vi "acquireVolumeAndFindNeurons.vi"   [LabVIEW 2017]
uses:
  globalUtilities.vi
  globalDevices.vi
  <userlib>/Hamamatsu Video Capture/tm_getframe16_40.vi
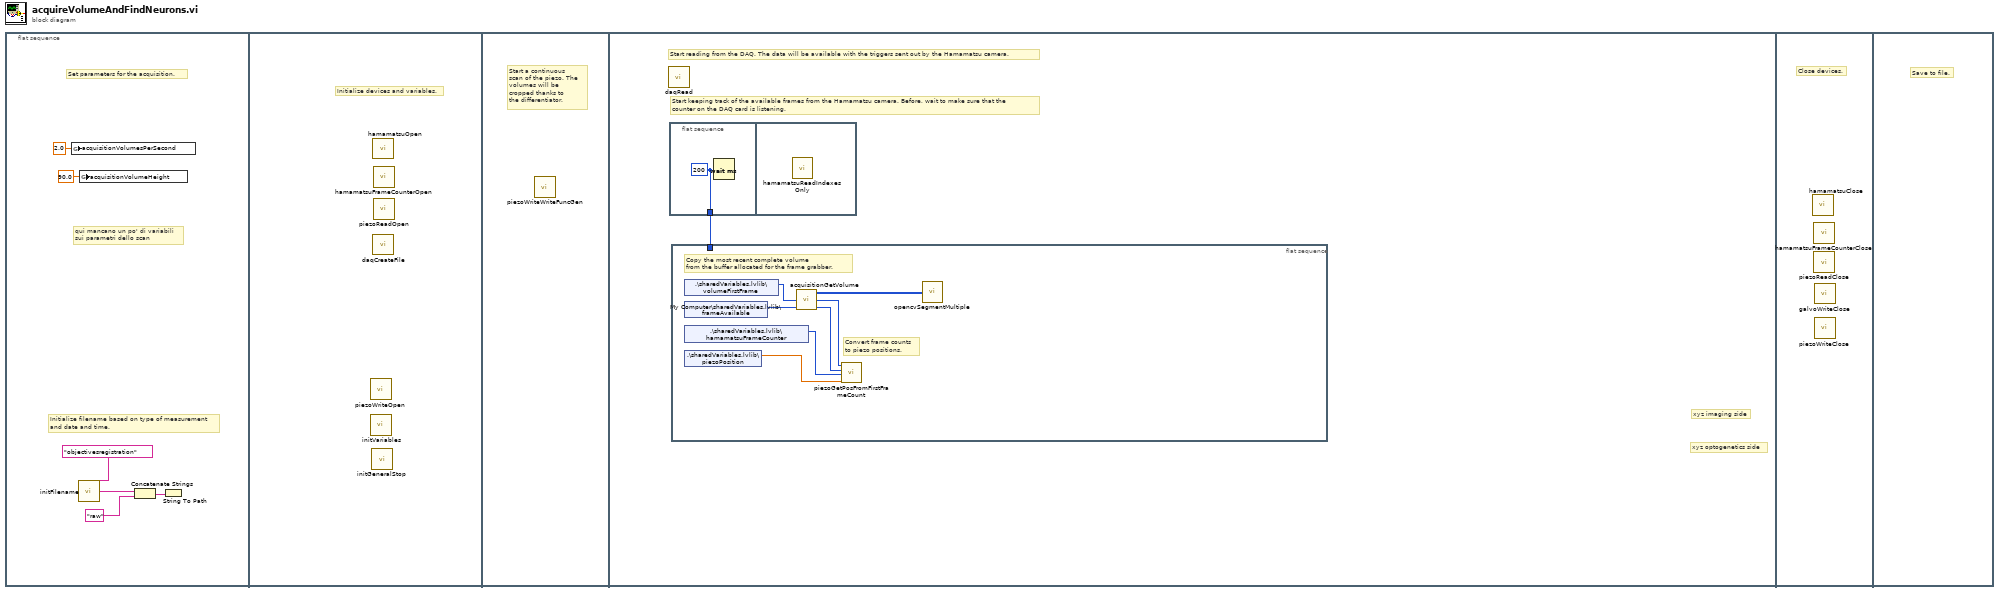
[diagram p0: block diagram]
diagram:
  n1 = flat-sequence {
    frame #0 {
      # "Initialize filename based on type of measurement\nand date and time."
      # "qui mancano un po' di variabili\nsui parametri dello scan"
      # "Set parameters for the acquisition."
      n2 = global write "globalUtilities.vi" "acquisitionVolumesPerSecond"(2.0 ("acquisitionVolumesPerSecond")) -> ()
      n3 = call "initFilename.vi"("Experiment type"="objectivesregistration") -> ("folder name"=w1:string)  [unwired: 1 in]
      n4 = global write "globalUtilities.vi" "acquisitionVolumeHeight"(90.0 ("acquisitionVolumeHeight")) -> ()
      n5 = Concatenate Strings(w1, "raw") -> (w2:string)
      n6 = String To Path(string=w2) -> ()  [unwired: 1 out]
    }
    frame #1 {
      # "Initialize devices and variables."
      n7 = call "piezoWriteOpen.vi"() -> ()  [unwired: 2 in]
      n8 = call "initVariables.vi"() -> ()  [unwired: 12 in]
      n9 = call "initGeneralStop.vi"() -> ()  [unwired: 1 in]
      n10 = call "hamamatsuOpen.vi"() -> ()  [unwired: 4 out]
      n11 = call "daqCreateFile.vi"() -> ()  [unwired: 12 in]
      n12 = call "hamamatsuFrameCounterOpen.vi"() -> ()  [unwired: 12 in]
      n13 = call "piezoReadOpen.vi"() -> ()  [unwired: 6 in]
    }
    frame #2 {
      # "Start a continuous\nscan of the piezo. The \nvolumes will be\ncropped thanks to\nthe differentiator."
      n14 = call "piezoWriteWriteFuncGen.vi"() -> ()  [unwired: 12 in]
    }
    frame #3 {
      # "Start keeping track of the available frames from the Hamamatsu camera. Before, wait to make sure that the\ncounter on the DAQ card is listening."
      # "Start reading from the DAQ. The data will be available with the triggers sent out by the Hamamatsu camera."
      # "xyz optogenetics side"
      # "xyz imaging side"
      n15 = call "daqRead.vi"() -> ()  [unwired: 3 in]
      n16 = flat-sequence {
        tunnel: [w15] -> w7
        frame #0 {
          w15 = u32 200 ("milliseconds to wait")
          n17 = Wait (ms)(milliseconds to wait=w15) -> ()  [unwired: 1 out]
        }
        frame #1 {
          n18 = call "hamamatsuReadIndexesOnly.vi"() -> ()  [unwired: 12 in]
        }
      }
      n19 = flat-sequence {
        tunnel: w7 -> [_]
        frame #0 {
          # "Convert frame counts\nto piezo positions."
          # "Copy the most recent complete volume\nfrom the buffer allocated for the frame grabber."
          n20 = shared-variable ".\\sharedVariables.lvlib\\volumeFirstFrame"() -> (w14:u32[])  [unwired: 1 in, 1 out]
          n21 = shared-variable ".\\sharedVariables.lvlib\\piezoPosition"() -> (w9:dbl[])  [unwired: 1 in, 1 out]
          n22 = shared-variable "My Computer\\sharedVariables.lvlib\\frameAvailable"() -> (w13:i32[])  [unwired: 1 in, 1 out]
          n23 = shared-variable ".\\sharedVariables.lvlib\\hamamatsuFrameCounter"() -> (w10:u32[])  [unwired: 1 in, 1 out]
          n24 = call "acquisitionGetVolume.vi"("frameAvailable"=w13, "volumeFirstFrame"=w14) -> ("numberOfFrames"=w11:u32, "absoluteCountFirstFrame"=w12:u32, "volume out"=w8:u16[][][])  [unwired: 1 in]
          n25 = call "piezoGetPosFromFirstFrameCount.vi"("piezoPosition"=w9, "hamamatsuFrameCounter"=w10, "numberOfFrames"=w11, "firstFrameCount"=w12) -> ()  [unwired: 2 in, 1 out]
          n26 = call "opencvSegmentMultiple.vi"("ImgIn"=w8) -> ()  [unwired: 2 out]
        }
      }
    }
    frame #4 {
      # "Close devices."
      n27 = call "hamamatsuClose.vi"() -> ()  [unwired: 1 out]
      n28 = call "hamamatsuFrameCounterClose.vi"() -> ()  [unwired: 12 in]
      n29 = call "piezoReadClose.vi"() -> ()  [unwired: 1 in]
      n30 = call "galvoWriteClose.vi"() -> ()  [unwired: 12 in]
      n31 = call "piezoWriteClose.vi"() -> ()  [unwired: 1 in]
    }
    frame #5 {
      # "Save to file."
    }
  }
